vi "test - #111.vi"(8 "error in (no error)":errorcluster, 11 "TestCase in":refnum<class "testcase-Supported-Datatype.lvclass">) -> (0 "error out":errorcluster, 3 "TestCase out":refnum<class "testcase-Supported-Datatype.lvclass">)   [LabVIEW 2017, in "testcase-Supported-Datatype.lvclass"]
uses:
  testcase-Supported-Datatype.lvclass
  1c8d65e4-54f0-4c15-bd12-dca4c41a2794.vi
  014bc8cd-b6f1-4d2f-837f-d94319000663.vi
  91b750c6-eb8b-4ec9-8eae-665cf872a29a.vi
  <vilib>/addons/_JKI Toolkits/VI Tester/TestCase.llb/TestCase.lvclass
  addons/API-String-Arugments-Support/API String Arguments Support.lvlib
  C:/Program Files (x86)/National Instruments/LabVIEW 2017/vi.lib/addons/_JKI Toolkits/VI Tester/TestCase.llb/TestCase.lvclass
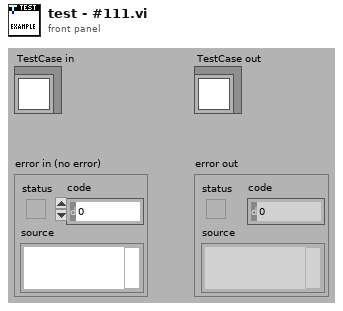
[diagram p1: front panel]
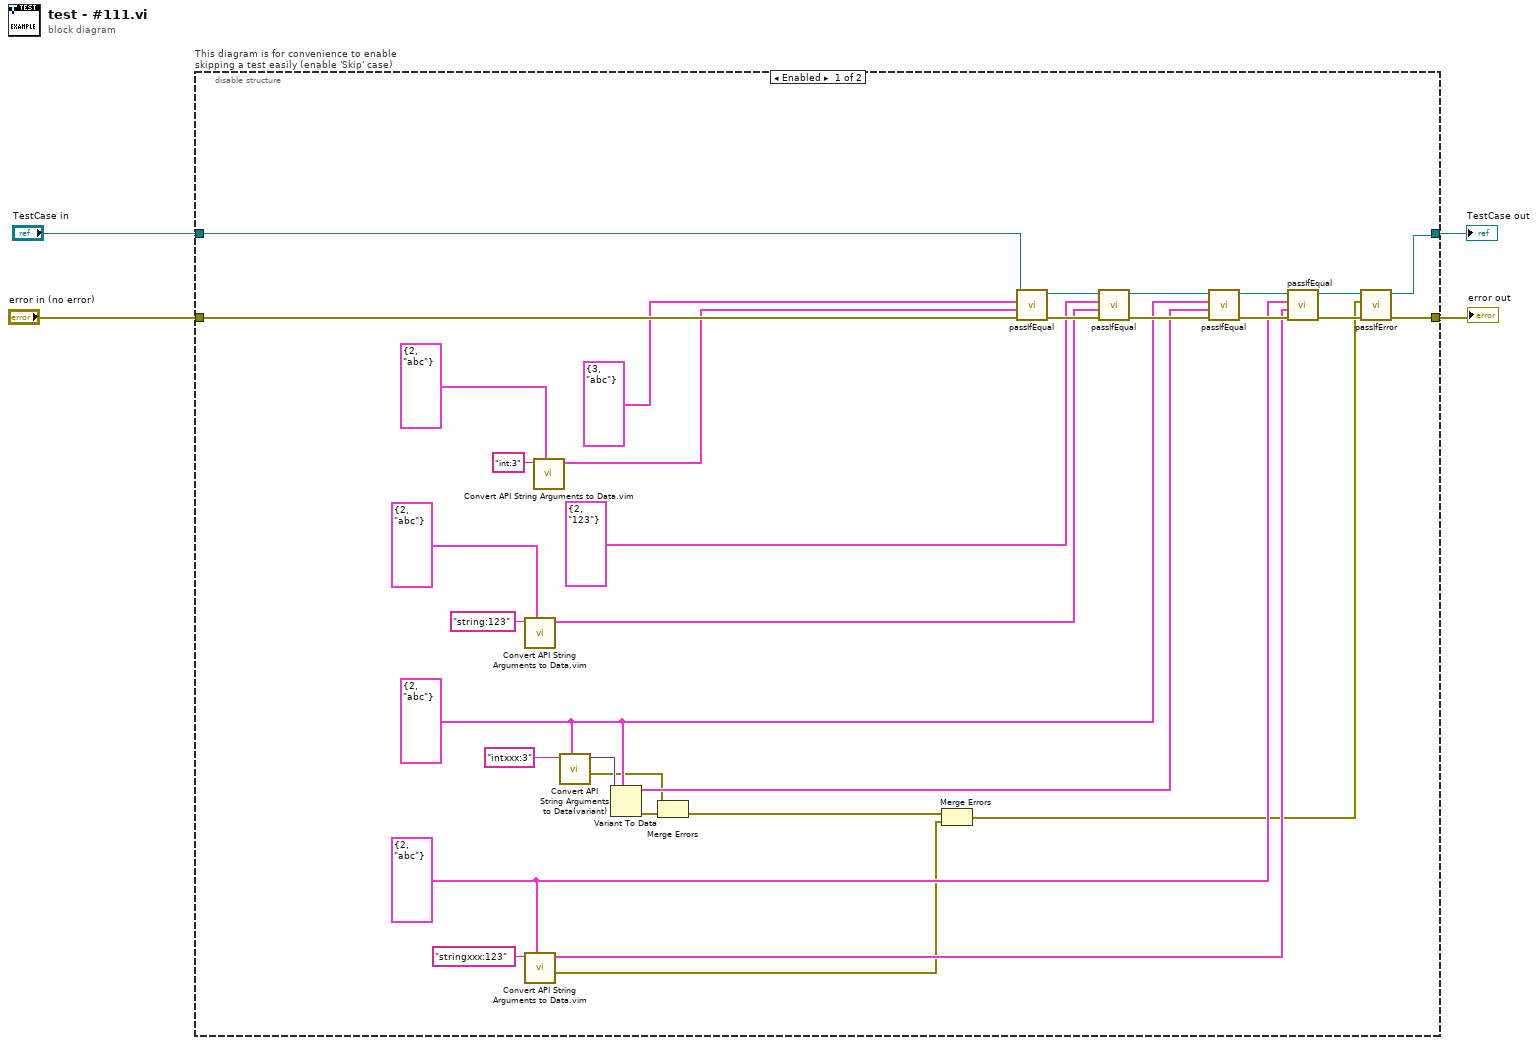
[diagram p0: block diagram]
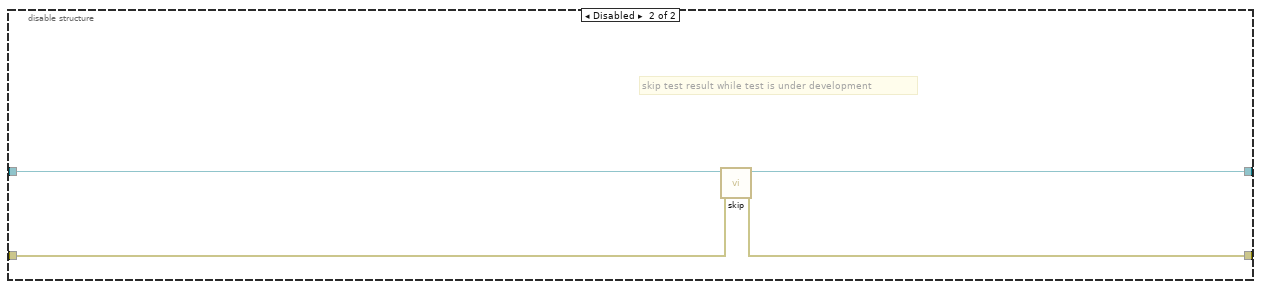
[diagram p2: hidden frame]
diagram:
  n1 = disable-structure "This diagram is for convenience to enable skipping a test easily (enable 'Skip' case)" shown="Enabled" {
    disable-tunnel: "TestCase in" -> [w36 w40]
    disable-tunnel: [w14 w38] -> w1
    disable-tunnel: [w17 w39] -> w3
    disable-tunnel: "error in (no error)" -> [w35 w37]
    frame Enabled {
      w19 = cluster{"int":i32, "string":string} {"int"=2, "string"="abc"}
      w10 = cluster{"int":i32, "string":string} {"int"=2, "string"="abc"}
      n2 = call "Convert API String Arguments to Data.vim"("Reference Type"=cluster{"int":i32, "string":string} {"int"=2, "string"="abc"}, "API String"="string:123") -> ("Data"=w21:cluster{"int":i32, "string":string})  [unwired: 6 in, 1 out]
      n3 = call "Convert API String Arguments to Data.vim"("Reference Type"=w19, "API String"="stringxxx:123") -> ("error out"=w12:errorcluster, "Data"=w18:cluster{"int":i32, "string":string})  [unwired: 6 in]
      n4 = call "Convert API String Arguments to Data.vim"("Reference Type"=cluster{"int":i32, "string":string} {"int"=2, "string"="abc"}, "API String"="int:3") -> ("Data"=w26:cluster{"int":i32, "string":string})  [unwired: 6 in, 1 out]
      n5 = call "Convert API String Arguments to Data(variant).vi"("Type"=w10, "String"="intxxx:3" ("API String")) -> ("error"=w5:errorcluster, "Data"=w11:variant)  [unwired: 8 in]
      n6 = Variant To Data(type=w10, Variant=w11) -> (data=w9:cluster{"int":i32, "string":string}, error out=w8:errorcluster)  [unwired: 1 in]
      n7 = Merge Errors(w5, w8) -> (w6:errorcluster)
      n8 = Merge Errors(w6, w12) -> (w13:errorcluster)
      n9 = call-dynamic "passIfEqual.vi"("error in (no error)"=w35, "y"=w26, "x"=cluster{"int":i32, "string":string} {"int"=3, "string"="abc"}, "TestCase in"=w36) -> ("error out"=w31:errorcluster, "TestCase out"=w34:refnum<class "testcase-Supported-Datatype.lvclass">)  [unwired: 6 in]
      n10 = call-dynamic "passIfEqual.vi"("error in (no error)"=w31, "y"=w21, "x"=cluster{"int":i32, "string":string} {"int"=2, "string"="123"}, "TestCase in"=w34) -> ("error out"=w32:errorcluster, "TestCase out"=w33:refnum<class "testcase-Supported-Datatype.lvclass">)  [unwired: 6 in]
      n11 = call-dynamic "passIfEqual.vi"("error in (no error)"=w32, "y"=w9, "x"=w10, "TestCase in"=w33) -> ("error out"=w30:errorcluster, "TestCase out"=w29:refnum<class "testcase-Supported-Datatype.lvclass">)  [unwired: 6 in]
      n12 = call-dynamic "passIfEqual.vi"("error in (no error)"=w30, "y"=w18, "x"=w19, "TestCase in"=w29) -> ("error out"=w16:errorcluster, "TestCase out"=w15:refnum<class "testcase-Supported-Datatype.lvclass">)  [unwired: 6 in]
      n13 = call-dynamic "passIfError.vi"("error in (no error)"=w16, "error"=w13, "TestCase in"=w15) -> ("error out"=w17:errorcluster, "TestCase out"=w14:refnum<class "testcase-Supported-Datatype.lvclass">)  [unwired: 7 in]
    }
    frame Disabled {
      # "skip test result while test is under development"
      n14 = call <vilib>:"skip.vi"("error in (no error)"=w37, "TestCase in"=w40) -> ("error out"=w39:errorcluster, "TestCase out"=w38:refnum<class "testcase-Supported-Datatype.lvclass">)  [unwired: 8 in]
    }
  }
  "error out" <- w3
  "TestCase out" <- w1
